vi "Parse Bookmarks.vi"(8 "error in (no error)":errorcluster {"code" format="Error %.0f"}, 10 "VI Reference":refnum<vi>, 11 "VIDoc Parser In":refnum<class "VIDoc Parser.lvclass">) -> (0 "error out":errorcluster {"code" format="Error %.0f"}, 2 "Bookmarked?":bool, 3 "VIDoc Parser Out":refnum<class "VIDoc Parser.lvclass">)   [LabVIEW 2023, in "VIDoc Parsing.lvlib" / "VIDoc Parser.lvclass"]
uses:
  VIDoc Parser.lvclass
  VIDoc Parser.lvclass/VIDoc Parser.ctl
  GUI Documentation/GUI Documentation.lvclass
  <vilib>/Utility/miscctls.llb/LVMapReplaceAction.ctl
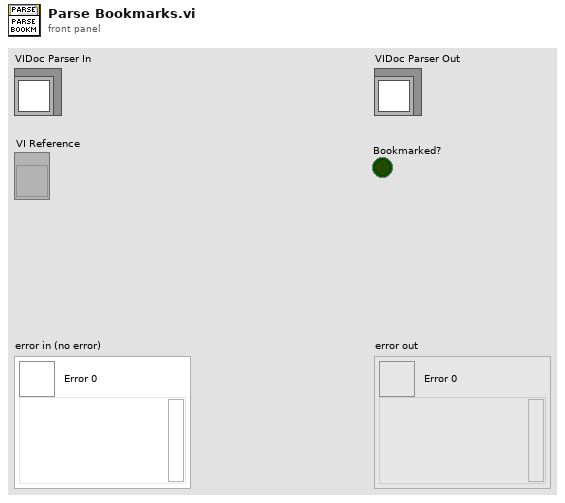
[diagram p1: front panel]
types:
  T1 = typedef "LVBookmarkInfoTypeDef.ctl" = cluster{"Bookmark Reference":u32, "Bookmark Tag":string, "Label Text":string}[]
  T2 = typedef "VIDoc Parsing.lvlib/Parser Settings.lvclass/Parser Settings Cluster.ctl" = cluster{"Draw Controls":T3, "Max Control Recursion Depth":i32, "Bookmarks Map":map{string, string[]}}
  T3 = typedef "VIDoc Parsing.lvlib/Parser Settings.lvclass/Draw Controls Cluster.ctl" = cluster{"Subpanels":bool, "Tabs":bool, "TypeDefs":bool, "Error Clusters":T4, "DVRs":T4, "Queues & Notifiers":T4}
  T4 = typedef "VIDoc Parsing.lvlib/Parser Settings.lvclass/Draw Option Enum.ctl" = enum16{"Ignore", "Draw", "Draw + Contents"}
  T5 = map{string, refnum<class "GUI Documentation.lvclass">[]}
  T6 = typedef "LVMapReplaceAction.ctl" = enum32{"Modify Entry only if found", "Add or Modify Entry", "Delete Entry"}
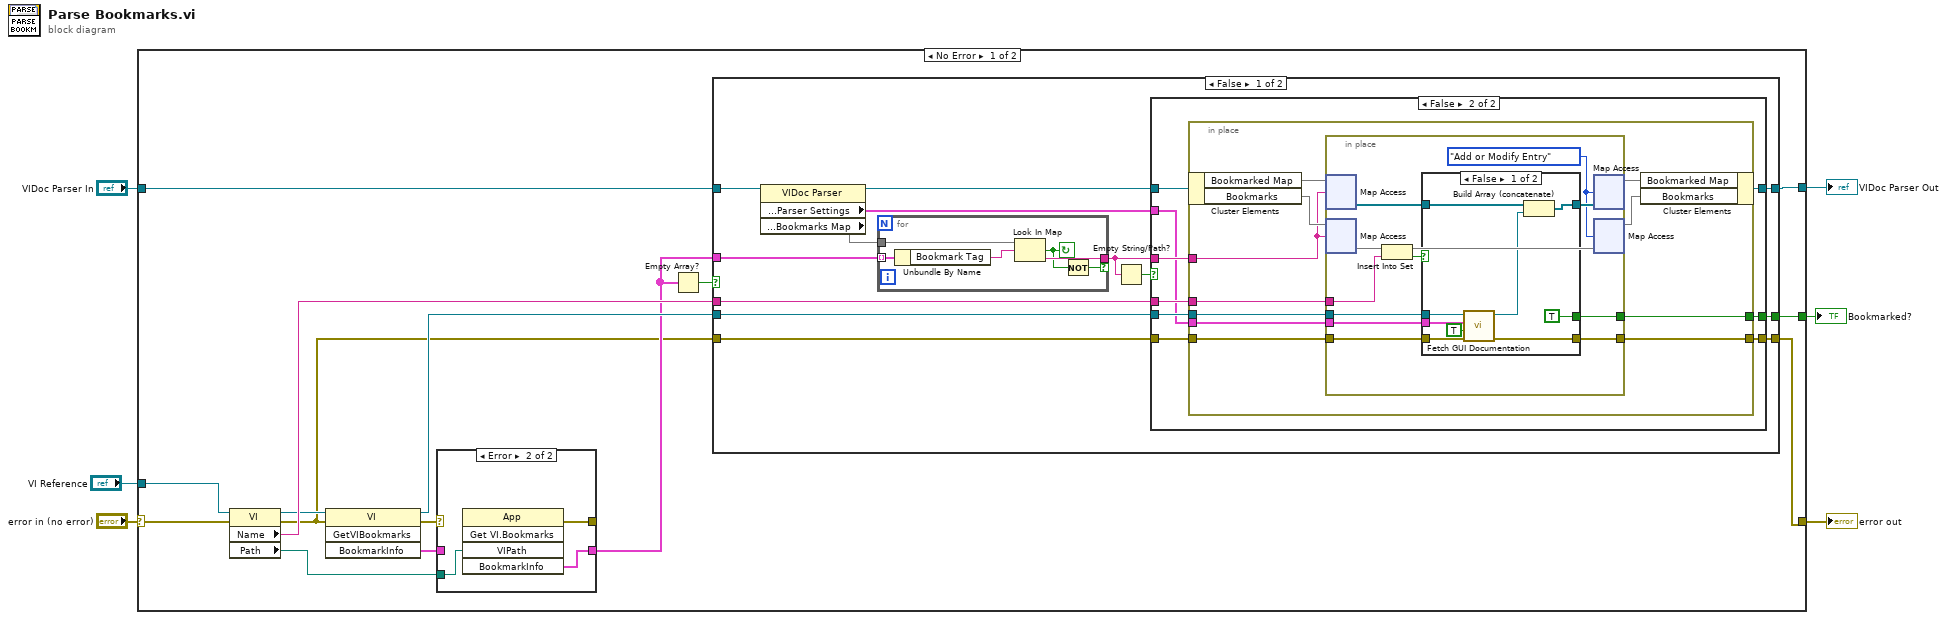
[diagram p0: block diagram]
diagram:
  n1 = case shown="No Error" "error in (no error)" {
    selector: "error in (no error)" -> [w19 w94]
    tunnel: [w17 w94] -> w5
    tunnel: [w20 w93] -> w3
    tunnel: "VIDoc Parser In" -> [w14 w93]
    tunnel: "VI Reference" -> [w18 _]
    tunnel: [w16 _] -> w1
    frame No Error {
      n2 = property class="VI"(reference=w18, error in=w19) -> (reference out=w11:refnum<vi>, error out=w8:errorcluster, "Name"=w15:string, "Path"=w7:path)
      n3 = invoke class="VI" method="GetVIBookmarks"(reference=w11, error in=w8) -> (reference out=w10:refnum<vi>, error out=w12:errorcluster, "BookmarkInfo"=w13:T1)  [unwired: 2 in, 1 out]
      n4 = case shown="Error" w12 {
        selector: w12 -> [w22 _]
        tunnel: w13 -> [w23 _]
        tunnel: [w23 w25] -> w9
        tunnel: [w22 w26] -> _
        tunnel: w7 -> [_ w24]
        frame No Error {
        }
        frame Error {
          n5 = invoke class="App" method="Get VI.Bookmarks"("VIPath"=w24) -> (error out=w26:errorcluster, "BookmarkInfo"=w25:T1)  [unwired: 4 in, 3 out]
        }
      }
      n6 = Empty Array?(array=w9) -> (empty?=w21:bool)
      n7 = case shown="False" w21 {
        tunnel: w9 -> [w38 _]
        tunnel: w14 -> [w30 w91]
        tunnel: [w39 w91] -> w20
        tunnel: w15 -> [w37 _]
        tunnel: w10 -> [w36 _]
        tunnel: w8 -> [w35 w92]
        tunnel: [w34 w92] -> w17
        tunnel: [w33 _] -> w16
        frame False {
          n8 = property class="VIDoc Parser"(reference=w30) -> (reference out=w29:refnum<class "VIDoc Parser.lvclass">, "Properties:Settings:Parser Settings"=w32:T2, "Properties:Settings:Bookmarks Map"=w31:map{string, string})  [unwired: 1 in, 1 out]
          n9 = for {
            tunnel: w38 -> [w45] mode=indexing
            tunnel: w31 -> [w44]
            tunnel: [w42] -> w28 if=w40
            stop <- w41 continue-if-true
            n10 = Unbundle By Name(w45) -> ("Bookmark Tag"=w43:string)
            n11 = Look In Map(map=w44, key=w43) -> (key not found?=w41:bool, value=w42:string)  [unwired: 1 in]
            n12 = Not(x=w41) -> (.not. x?=w40:bool)
          }
          n13 = Empty String/Path?(string/path=w28) -> (empty?=w27:bool)
          n14 = case shown="False" w27 {
            tunnel: w29 -> [w47 w56]
            tunnel: [w47 w55] -> w39
            tunnel: w32 -> [_ w51]
            tunnel: w37 -> [_ w53]
            tunnel: w36 -> [_ w52]
            tunnel: w35 -> [w46 w50]
            tunnel: [w46 w49] -> w34
            tunnel: [_ w48] -> w33
            tunnel: w28 -> [_ w54]
            frame True {
            }
            frame False {
              n15 = in-place "In Place Element Structure" {
                in-place-border: w54 -> [w65]
                in-place-border: w53 -> [w64]
                in-place-border: w52 -> [w63]
                in-place-border: w51 -> [w62]
                in-place-border: w50 -> [w61]
                in-place-border: [w60] -> w49
                in-place-border: [w57] -> w48
                n16 = in-place-cluster #1(w56) -> ("Bookmarked Map"=w67:T5, "Bookmarks"=w66:map{string, set{string}})
                n17 = in-place "In Place Element Structure" {
                  in-place-border: w64 -> [w76]
                  in-place-border: w63 -> [w73]
                  in-place-border: w62 -> [w72]
                  in-place-border: w61 -> [w71]
                  in-place-border: [w70] -> w60
                  in-place-border: [w68] -> w57
                  w69 = LVMapReplaceAction."Add or Modify Entry" ("action")
                  n18 = in-place-map #2(w67, w65) -> (w79:refnum<class "GUI Documentation.lvclass">[])  [unwired: 1 in, 1 out]
                  n19 = in-place-map #3(w66, w65) -> (w77:set{string})  [unwired: 1 in, 1 out]
                  n20 = Insert Into Set(10:w76, 11:w77) -> (2:w74:bool, 3:w75:set{string})
                  n21 = case shown="False" w74 {
                    tunnel: w79 -> [w87 w90]
                    tunnel: [w86 w90] -> w78
                    tunnel: w73 -> [w84 _]
                    tunnel: w72 -> [w83 _]
                    tunnel: w71 -> [w82 w89]
                    tunnel: [w81 w89] -> w70
                    tunnel: [TRUE _] -> w68
                    frame False {
                      n22 = call "Fetch GUI Documentation.vi"("error in (no error)"=w82, "Fetch Controls?"=TRUE, "Parser Settings"=w83, "VI Reference"=w84) -> ("error out"=w81:errorcluster, "GUI Documentation Out"=w85:refnum<class "GUI Documentation.lvclass">)  [unwired: 6 in]
                      n23 = Build Array (concatenate)(w87, w85) -> (w86:refnum<class "GUI Documentation.lvclass">[])
                    }
                    frame True {
                    }
                  }
                  n24 = in-place-map #2(w78, w69) -> (w59:T5)  [unwired: 2 out]
                  n25 = in-place-map #3(w75, w69) -> (w58:map{string, set{string}})  [unwired: 2 out]
                }
                n26 = in-place-cluster #1("Bookmarked Map"=w59, "Bookmarks"=w58) -> (w55:refnum<class "VIDoc Parser.lvclass">)
              }
            }
          }
        }
        frame True {
        }
      }
    }
    frame Error {
    }
  }
  "error out" <- w5
  "VIDoc Parser Out" <- w3
  "Bookmarked?" <- w1
